vi "main.vi"() -> ()   [LabVIEW 2025, in "Full Featured MCP Server.lvlib"]
doc: "This example demonstrates all features of the MCP Server toolkit with a demo-stock-broker. It has multiple stocks that have different prices and range. Multiple tools to retrieve stock prices or buy stocks. It also has some prompt templates and a resource with a \"power-prompt\" to enable better responses."
uses:
  Full Featured MCP Server.lvlib
  Server FGV Modes.ctl
  Get Owned Stocks.vi
  Buy Stock.vi
  Get History Chart.vi
  Get Stock Names.vi
  Get Stock Prices.vi
  Get Wallet.vi
  Buy Any.vi
  Find Best Trending Stock.vi
  <vilib>/jgoebel/LabVIEW MCP Server SDK/MCP Server.lvlib
panel:
  out "MCP Log":string
  out "Stock Prices":dbl[][](graph)
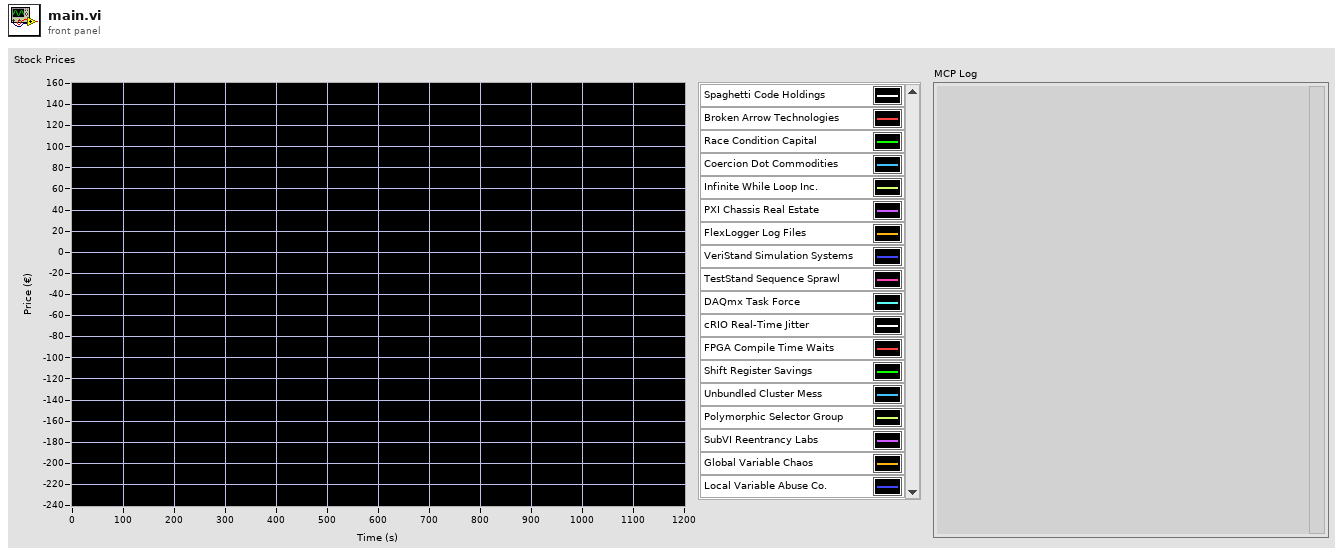
[diagram p1: front panel]
types:
  T1 = typedef "Full Featured MCP Server.lvlib/Server FGV Modes.ctl" = enum16{"Update Stocks", "Buy Stock", "Get All", "Init"}
  T2 = typedef "Full Featured MCP Server.lvlib/Server Data.ctl" = cluster{"Stocks Prices":dbl[][], "Owned Stocks":i32[], "Stock Names":string[], "Wallet":dbl, "Fluctuation":dbl, "Stock Trends":dbl[]}
  T3 = typedef "MCP Server.lvlib/User Events.ctl" = cluster{"onError":refnum<user-event>, "onLog":refnum<user-event>, "onConnect":refnum<user-event>, "onToolsList":refnum<user-event>, "onToolsCall":refnum<user-event>, "onNotification":refnum<user-event>, "onTool":refnum<user-event>, "onRpc":refnum<user-event>}
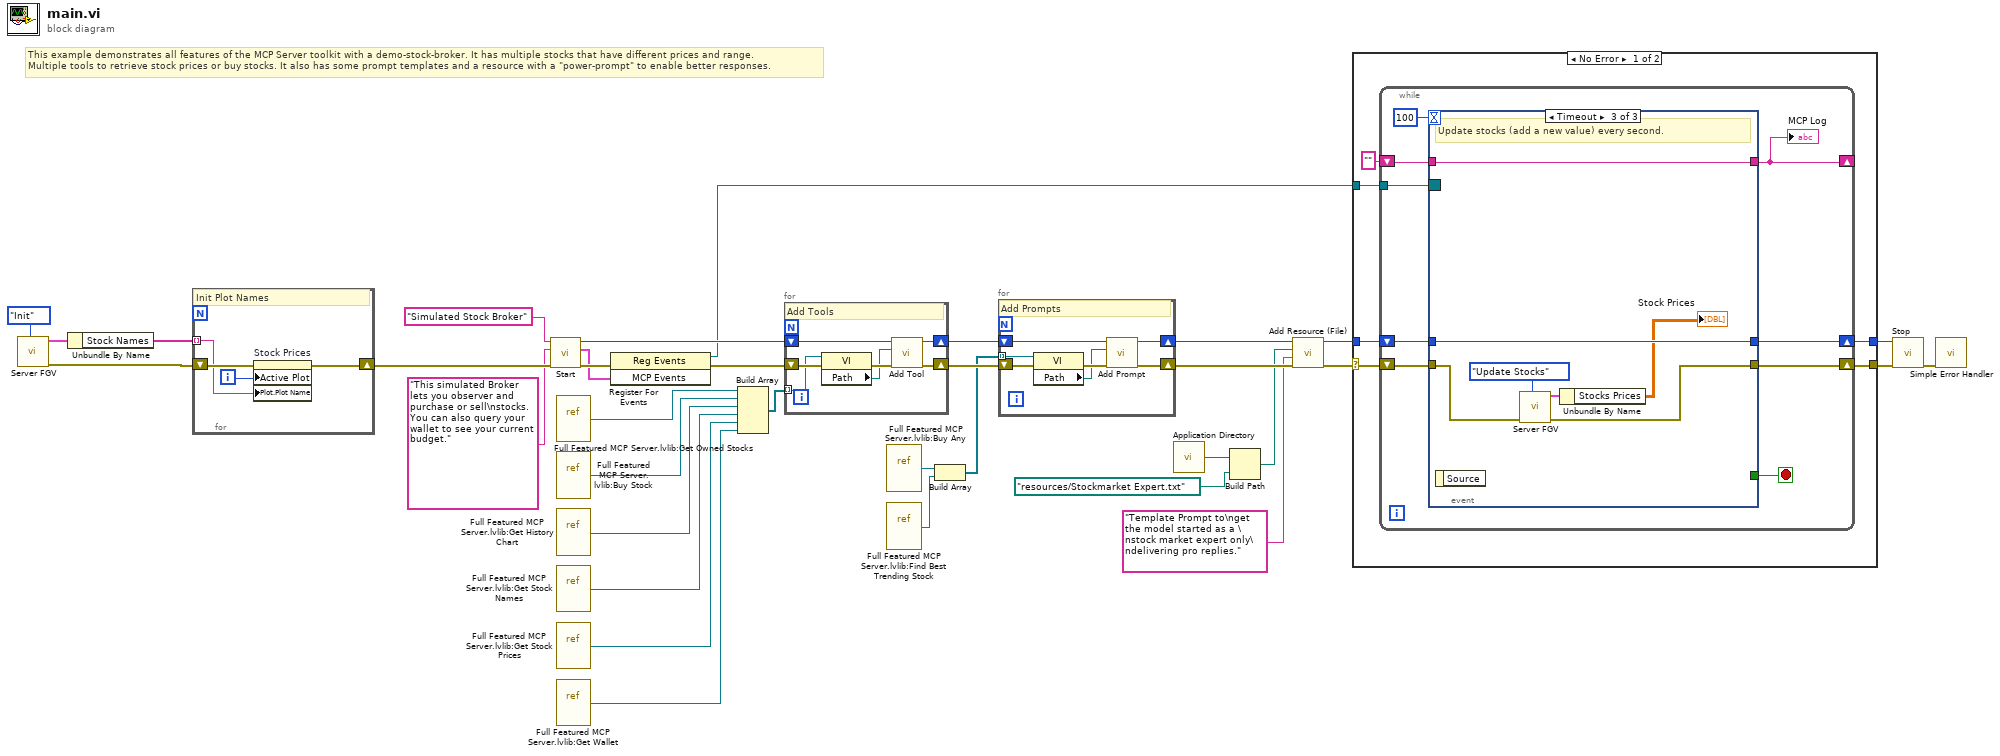
[diagram p0: block diagram]
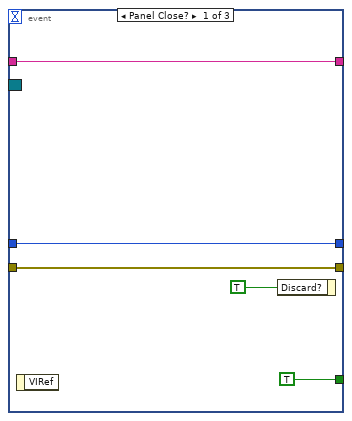
[diagram p2: hidden frame]
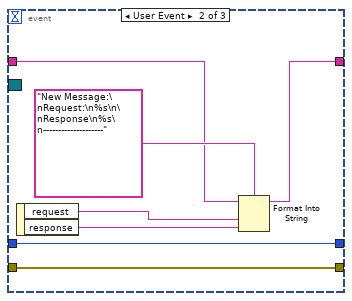
[diagram p3: hidden frame]
diagram:
  # "This example demonstrates all features of the MCP Server toolkit with a demo-stock-broker. It has multiple stocks that have different prices and range.\nMultiple tools to retrieve stock prices or buy stocks. It also has some prompt templates and a resource with a \"power-prompt\" to enable better responses."
  n1 = call "Server FGV.vi"("Mode (Get All)"=Server_FGV_Modes."Init") -> ("error out"=w13:errorcluster, "Full Features MCP Server Data"=w11:T2)  [unwired: 8 in, 1 out]
  n2 = Unbundle By Name(w11) -> ("Stock Names"=w10:string[])
  n3 = for {
    shift-right: [w38] -> w12
    shift-left: w13 -> [w39]
    tunnel: w10 -> [w36] mode=indexing
    i -> [w37]
    # "Init Plot Names"
    n4 = property on="Stock Prices" class="WFGraph (strict)"(error in=w39, "Active Plot"=w37, "Plot.Plot Name"=w36) -> (error out=w38:errorcluster)  [unwired: 1 in, 1 out]
  }
  n5 = call <vilib>:"Start.vi"("error in (no error)"=w12, "Description"="This simulated Broker lets you observer and purchase or sell\nstocks. You can also query your wallet to see your current budget.", "Name"="Simulated Stock Broker") -> ("error out"=w34:errorcluster, "MCP Events"=w24:T3, "id out"=w35:i32)  [unwired: 6 in]
  n6 = vi-ref "Full Featured MCP Server.lvlib:Get Owned Stocks.vi"() -> (w22:refnum<vi>)
  n7 = vi-ref "Full Featured MCP Server.lvlib:Buy Stock.vi"() -> (w18:refnum<vi>)
  n8 = vi-ref "Full Featured MCP Server.lvlib:Get History Chart.vi"() -> (w17:refnum<vi>)
  n9 = vi-ref "Full Featured MCP Server.lvlib:Get Stock Names.vi"() -> (w16:refnum<vi>)
  n10 = vi-ref "Full Featured MCP Server.lvlib:Get Stock Prices.vi"() -> (w15:refnum<vi>)
  n11 = vi-ref "Full Featured MCP Server.lvlib:Get Wallet.vi"() -> (w14:refnum<vi>)
  n12 = register-events(error in=w34, w24) -> (reference out=w23:refnum<event-registration>, error out=w25:errorcluster)  [unwired: 1 in]
  n13 = Build Array(w22, w18, w17, w16, w15, w14) -> (w21:refnum<vi>[])
  n14 = for {
    tunnel: w21 -> [w41] mode=indexing
    shift-right: [w45] -> w33
    shift-left: w35 -> [w46]
    shift-right: [w44] -> w32
    shift-left: w25 -> [w43]
    # "Add Tools"
    n15 = property class="VI"(reference=w41, error in=w43) -> (error out=w42:errorcluster, "Path"=w40:path)  [unwired: 1 out]
    n16 = call <vilib>:"Add Tool.vi"("error in (no error)"=w42, "vi path"=w40, "id"=w46) -> ("error out"=w44:errorcluster, "id out"=w45:i32)  [unwired: 7 in]
  }
  n17 = vi-ref "Full Featured MCP Server.lvlib:Buy Any.vi"() -> (w7:refnum<vi>)
  n18 = vi-ref "Full Featured MCP Server.lvlib:Find Best Trending Stock.vi"() -> (w5:refnum<vi>)
  n19 = Build Array(w7, w5) -> (w6:refnum<vi>[])
  n20 = for {
    tunnel: w6 -> [w48] mode=indexing
    shift-right: [w51] -> w31
    shift-left: w33 -> [w53]
    shift-right: [w50] -> w30
    shift-left: w32 -> [w52]
    # "Add Prompts"
    n21 = property class="VI"(reference=w48, error in=w52) -> (error out=w49:errorcluster, "Path"=w47:path)  [unwired: 1 out]
    n22 = call <vilib>:"Add Prompt.vi"("error in (no error)"=w49, "vi path"=w47, "server id"=w53) -> ("error out"=w50:errorcluster, "server id out"=w51:i32)  [unwired: 7 in]
  }
  n23 = call <vilib>:"Application Directory.vi"() -> ("Application Directory"=w3:path)
  n24 = Build Path(base path=w3, name or relative path=path "resources/Stockmarket Expert.txt") -> (appended path=w1:path)
  n25 = call <vilib>:"Add Resource (File).vi"("error in (no error)"=w30, "description"="Template Prompt to\nget the model started as a \nstock market expert only\ndelivering pro replies.", "file path"=w1, "server id"=w31) -> ("error out"=w19:errorcluster, "server id out"=w29:i32)  [unwired: 6 in]
  n26 = case shown="No Error" w19 {
    selector: w19 -> [w56 w89]
    tunnel: w29 -> [w59 w88]
    tunnel: [w58 w88] -> w28
    tunnel: [w57 w89] -> w27
    tunnel: w23 -> [w55 _]
    frame No Error {
      n27 = while {
        shift-right: [w66] -> w57
        shift-left: w56 -> [w67]
        shift-right: [w64] -> w58
        shift-left: w59 -> [w65]
        tunnel: w55 -> [w63]
        shift-right: [w61] -> _
        shift-left: "" -> [w60]
        stop <- w68 stop-if-true
        n28 = event shown="[2] Timeout" {
          selector: w63 -> [_ _ _]
          dyn-events: _ -> [_ _ _]
          timeout: 100 -> [_ _ _]
          tunnel: [TRUE _ _] -> w68
          tunnel: [w71 w80 w85] -> w66
          tunnel: w67 -> [w71 w80 w87]
          tunnel: w65 -> [w70 w79 w86]
          tunnel: [w70 w79 w86] -> w64
          tunnel: [w69 w75 w81] -> w61
          tunnel: w60 -> [w69 w74 w81]
          event Panel Close? {
            n29 = event-data() -> ()  [unwired: 1 in, 1 out]
            n30 = event-data("Discard?"=TRUE) -> ()  [unwired: 1 in, 1 out]
          }
          event User Event {
            n31 = event-data() -> ("request"=w77:string, "response"=w76:string)  [unwired: 1 in]
            n32 = Format Into String(format string="New Message:\nRequest:\n%s\n\nResponse\n%s\n--------------------", initial string=w74, w77, w76) -> (resulting string=w75:string)  [unwired: 1 in, 1 out]
          }
          event Timeout {
            # "Update stocks (add a new value) every second."
            n33 = event-data() -> ()  [unwired: 1 in, 1 out]
            n34 = call "Server FGV.vi"("Mode (Get All)"=Server_FGV_Modes."Update Stocks", "error in (no error)"=w87) -> ("error out"=w85:errorcluster, "Full Features MCP Server Data"=w83:T2)  [unwired: 7 in, 1 out]
            n35 = Unbundle By Name(w83) -> ("Stocks Prices"=→"Stock Prices":dbl[][])
          }
        }
        "MCP Log" <- w61
      }
    }
    frame Error {
    }
  }
  n36 = call <vilib>:"Stop.vi"("error in (no error)"=w27, "id"=w28) -> ("error out"=w26:errorcluster)  [unwired: 9 in]
  n37 = call <vilib>:"Simple Error Handler.vi"("error in (no error)"=w26) -> ()  [unwired: 4 in, 5 out]
